vi "Auto Play Path.vi"(7 "PID Constants":T1, 8 "Operation":T2, 9 "Auto Data":T14, 10 "Motors":T3 {"Radii (ft)"."Right Back Position" format="%.2f"; "Radii (ft)"."Right Front Position" format="%.2f"; "Radii (ft)"."Left Back Position" format="%.2f"; "Radii (ft)"."Left Front Position" format="%.2f"; "Pigeon2"."Type" items=["CAN"=352321536, "TalonSRX"=33554432]}) -> (0 "Auto Done?":bool)   [LabVIEW 2023]
uses:
  swerve/Type Definitions/Data/Robot Velocities.ctl
  swerve/Type Definitions/Hardware/Swerve Drives/(NEO-NEO-ThroughBore-Pigeon2) Swerve.ctl
  swerve/Type Definitions/Hardware/4 Motor Sets/(NEO & NEO 550) 4 Motor Set.ctl
  <vilib>/Rock Robotics/WPI/MotorControl/WPI_MotorControlDeviceRef.ctl
  <vilib>/Rock Robotics/WPI/MotorControl/WPI_MotorControlType.ctl
  <vilib>/Rock Robotics/SystemInterfaces/DIO/FPGA_DIOPWMChannel.ctl
  <vilib>/Rock Robotics/WPI/PWM/WPI_PWMDeadband.ctl
  <vilib>/Rock Robotics/SystemInterfaces/DIO/FPGA_DIOChannel.ctl
  <vilib>/Rock Robotics/WPI/ThirdParty/Phoenix-LabVIEW/Pigeon IMU/CTRE_PigeonIMU_DeviceRef.ctl
  <vilib>/Rock Robotics/WPI/ThirdParty/Phoenix-LabVIEW/Pigeon IMU/CTRE_PigeonIMU_ConnectionType.ctl
  swerve/Type Definitions/Data/Pod Positions.ctl
  Implementation/Drive Operations.ctl
  <vilib>/Platform/TimedLoop/XDataNode/timing_clust.ctl
  <vilib>/Platform/TimedLoop/XDataNode/nitl_modes.ctl
  <vilib>/Platform/TimedLoop/XDataNode/wakeup.ctl
  <vilib>/Rock Robotics/WPI/ThirdParty/REV Robotics/REVLib/Typedef/Spark MAX Control Type.ctl
  <vilib>/Rock Robotics/WPI/DriverStation/WPI_DriverStationRobotMode2.ctl
  c1434f1d-cc94-402a-bfa5-996335562ac8.vi
  Framework/Robot Global Data.vi
  <vilib>/Platform/TimedLoop/XDataNode/XDataNode.xnode
  <vilib>/Platform/TimedLoop/XDataNode/XDNodeRunTimeDep.lvlib
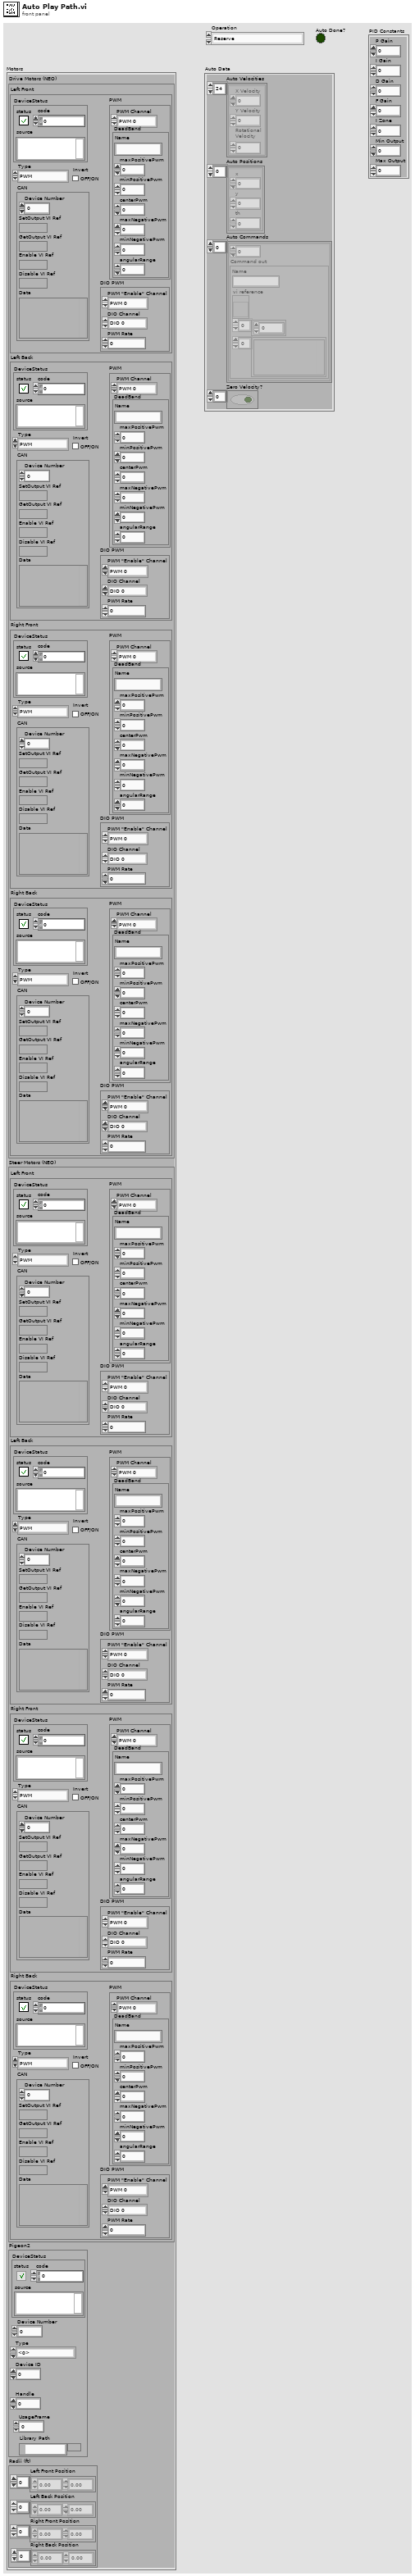
[diagram p1: front panel]
types:
  T1 = cluster{"P Gain":dbl, "I Gain":dbl, "D Gain":dbl, "F Gain":dbl, "I Zone":dbl, "Min Output":dbl, "Max Output":dbl}
  T2 = typedef "Drive Operations.ctl" = enum16{"Reserve", "Read Current", "Immediate", "Calibrate", "Reef Align", "Auto", "Old Reef Align"}
  T3 = typedef "(NEO-NEO-ThroughBore-Pigeon2) Swerve.ctl" = cluster{"Drive Motors (NEO)":T4, "Steer Motors (NEO)":T4, "Pigeon2":T10, "Radii (ft)":T12}
  T4 = typedef "(NEO & NEO 550) 4 Motor Set.ctl" = cluster{"Left Front":T5, "Left Back":T5, "Right Front":T5, "Right Back":T5}
  T5 = typedef "WPI_MotorControlDeviceRef.ctl" = cluster{"DeviceStatus":errorcluster, "Type":T6, "PWM":cluster{"PWM Channel":T7, "DeadBand":T8}, "CAN":cluster{"Device Number":u8, "SetOutput VI Ref":variant, "GetOutput VI Ref":variant, "Enable VI Ref":variant, "Disable VI Ref":variant, "Data":variant}, "Invert":bool, "DIO PWM":cluster{"PWM \"Enable\" Channel":T7, "DIOChannel":T9, "PWM Rate":dbl}}
  T6 = typedef "WPI_MotorControlType.ctl" = enum16{"PWM", "CAN", "DIO PWM"}
  T7 = typedef "FPGA_DIOPWMChannel.ctl" = enum8{"PWM 0", "PWM 1", "PWM 2", "PWM 3", "PWM 4", "PWM 5", "PWM 6", "PWM 7", "PWM 8", "PWM 9", "PWM MXP 0", "PWM MXP 1", "PWM MXP 2", "PWM MXP 3", "PWM MXP 4", "PWM MXP 5", "PWM MXP 6", "PWM MXP 7", "PWM MXP 8", "PWM MXP 9", "Invalid"}
  T8 = typedef "WPI_PWMDeadband.ctl" = cluster{"Name":string, "maxPositivePwm":i32, "minPositivePwm":i32, "centerPwm":i32, "maxNegativePwm":i32, "minNegativePwm":i32, "angularRange":u16}
  T9 = typedef "FPGA_DIOChannel.ctl" = enum8{"DIO 0", "DIO 1", "DIO 2", "DIO 3", "DIO 4", "DIO 5", "DIO 6", "DIO 7", "DIO 8", "DIO 9", "DIO MXP 0", "DIO MXP 1", "DIO MXP 2", "DIO MXP 3", "DIO MXP 4", "DIO MXP 5", "DIO MXP 6", "DIO MXP 7", "DIO MXP 8", "DIO MXP 9", "DIO MXP 10", "DIO MXP 11", "DIO MXP 12", "DIO MXP 13", "DIO MXP 14", "DIO MXP 15", "SPI Port CS1", "SPI Port CS2", "SPI Port CS3", "SPI Port MISO", "SPI Port MOSI", "Invalid"}
  T10 = typedef "CTRE_PigeonIMU_DeviceRef.ctl" = cluster{"DeviceStatus":errorcluster, "Device Number":u8, "Type":T11, "Device ID":u32, "Handle":u64, "UsageFrame":u32, "Library Path":path}
  T11 = typedef "CTRE_PigeonIMU_ConnectionType.ctl" = u32
  T12 = typedef "Pod Positions.ctl" = cluster{"Left Front Position":dbl[], "Left Back Position":dbl[], "Right Front Position":dbl[], "Right Back Position":dbl[]}
  T13 = typedef "Robot Velocities.ctl" = cluster{"X Velocity":dbl, "Y Velocity":dbl, "Rotational \nVelocity":dbl}
  T14 = cluster{"Auto Velocities":T13[], "Auto Positions":cluster{"x":dbl, "y":dbl, "th":dbl}[], "Auto Commands":cluster{dbl, "Command out":cluster{"Name":string, "vi reference":refnum<vi>, i32[], variant[]}}[], "Zero Velocity?":bool[]}
  T15 = cluster{"Time (s)":dbl, "Command out":cluster{"Name":string, "vi reference":refnum<vi>, i32[], variant[]}}
  T16 = typedef "Spark MAX Control Type.ctl" = enum16{"Percent VBus", "Voltage", "Velocity", "Position", "Smart Motion", "Current", "Smart Velocity", "MAXMotion Position", "MAXMotion Velocity"}
  T17 = cluster{"Left Front":dbl, "Left Back":dbl, "Right Front":dbl, "Right Back":dbl}
  T18 = typedef "XDNodeRunTimeDep.lvlib/timing_clust.ctl" = cluster{"Expected End [f-1]":u64, "Actual End [f-1]":u64, "Finished Late? [f-1]":bool, "Expected End [i-1]":u64, "Actual End [i-1]":u64, "Finished Late? [i-1]":bool, "Expected Start [i]":u64, "Actual Start [i]":u64, "Expected Start [f]":u64, "Actual Start [f]":u64, "Source Name":string, "Structure Name":string, "Period":i64, "Deadline":i64, "Offset":i64, "Start":i64, "Priority":i32, "Timeout":i32, "Mode":T19, "Wakeup Reason":T20, "Error":errorcluster, "Source Type":string, "Secondary Source Type":string, "Global End Time":u64, "Global Start Time":u64, "Frame Duration":u64, "Iteration Duration":u64, "Assigned CPU":i32, "I/O Scan Engine Mode":u32}
  T19 = typedef "XDNodeRunTimeDep.lvlib/nitl_modes.ctl" = enum32{"No Change", "Process missed periods, maintain original phase", "Discard missed periods, maintain original phase", "Process missed periods, ignore original phase", "Discard missed periods, ignore original phase"}
  T20 = typedef "XDNodeRunTimeDep.lvlib/wakeup.ctl" = enum32{"Normal", "Aborted", "Asynchronous wakeup", "Timing source error", "Timed loop error", "Timeout"}
  T21 = cluster{dbl, "Command out":cluster{"Name":string, "vi reference":refnum<vi>, i32[], variant[]}}[]
  T22 = typedef "WPI_DriverStationRobotMode2.ctl" = enum16{"Autonomous Disabled", "Autonomous Enabled", "Teleop Disabled", "Teleop Enabled", "Disconnected", "Finish", "Test Disabled", "Test Enabled", "Emergency Stopped"}
  T23 = cluster{"Field Centric":bool, "Reef Centric":bool}
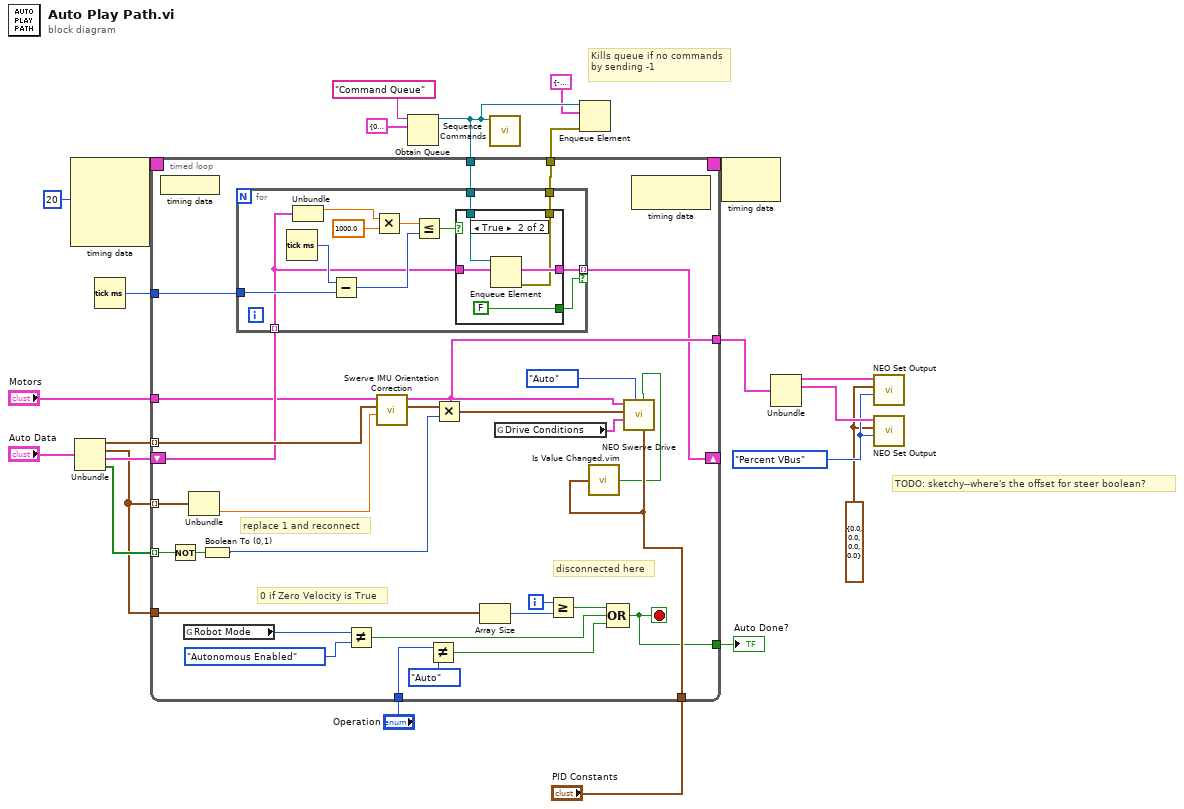
[diagram p0: block diagram]
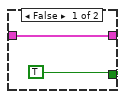
[diagram p2: hidden frame]
diagram:
  w8 = Spark_MAX_Control_Type."Percent VBus" ("Control Mode")
  w7 = T17 {"Left Front"=0.0, "Left Back"=0.0, "Right Front"=0.0, "Right Back"=0.0} ("Setpoints")
  # "TODO: sketchy--where's the offset for steer boolean?"
  # "Kills queue if no commands by sending -1"
  n1 = node-c288(i64 20 ("Period")) -> (w23:T18)  [unwired: 3 in]
  n2 = Unbundle("Auto Data") -> ("Auto Velocities"=w16:T13[], "Auto Positions"=w17:cluster{"x":dbl, "y":dbl, "th":dbl}[], "Auto Commands"=w19:T21, "Zero Velocity?"=w20:bool[])
  n3 = Tick Count (ms)() -> (millisecond timer value=w18:u32)
  n4 = Obtain Queue(name (unnamed)="Command Queue", element data type=T15 {"Time (s)"=0.0, "Command out"={"Name"="", "vi reference"=refnum, [], []}} ("element")) -> (queue out=w4:refnum<queue>)  [unwired: 3 in, 2 out]
  n5 = timed-loop {
    timing: w23 -> [_]
    timing-out: [_] -> w22
    tunnel: "Motors" -> [w39]
    tunnel: [w51] -> w6
    tunnel: w16 -> [w50] mode=indexing
    tunnel: w17 -> [w49] mode=indexing
    tunnel: w17 -> [w48]
    tunnel: w18 -> [w47]
    tunnel: w4 -> [w46]
    shift-right: [w45] -> _
    shift-left: w19 -> [w44]
    tunnel: w20 -> [w40] mode=indexing
    tunnel: [w29] -> w21
    tunnel: "Operation" -> [w38]
    tunnel: [w37] -> w3
    tunnel: "PID Constants" -> [w34]
    i -> [w52]
    stop <- w29 stop-if-true
    # "replace 1 and reconnect"
    # "disconnected here"
    # "0 if Zero Velocity is True"
    n6 = node-c288() -> ()  [unwired: 1 in]
    n7 = Not(x=w40) -> (.not. x?=w28:bool)
    n8 = global read "Robot Global Data.vi" "Robot Mode"() -> (w33:T22)
    n9 = Unbundle(w49) -> ("th"=w35:dbl)  [unwired: 2 out]
    n10 = Boolean To (0,1)(Boolean=w28) -> (0, 1=w27:i16)
    n11 = for {
      tunnel: w47 -> [w64]
      tunnel: w46 -> [w58]
      tunnel: w44 -> [w55] mode=indexing
      tunnel: [w57] -> w45 mode=indexing if=w56
      tunnel: [w54] -> w37
      n12 = Tick Count (ms)() -> (millisecond timer value=w65:u32)
      n13 = Unbundle(w55) -> (w63:dbl)  [unwired: 1 out]
      n14 = Subtract(x=w65, y=w64) -> (x-y=w60:u32)
      n15 = Multiply(x=w63, y=1000.0) -> (x*y=w61:dbl)
      n16 = Less Or Equal?(x=w61, y=w60) -> (x <= y?=w59:bool)
      n17 = case shown="True" w59 {
        tunnel: w58 -> [_ w71]
        tunnel: w55 -> [w66 w70]
        tunnel: [w66 w70] -> w57
        tunnel: [TRUE FALSE] -> w56
        tunnel: [_ w68] -> w54
        frame False {
        }
        frame True {
          n18 = Enqueue Element(queue=w71, element=w70) -> (error out=w68:errorcluster)  [unwired: 2 in, 2 out]
        }
      }
    }
    n19 = Not Equal?(x=w33, y=WPI_DriverStationRobotMode2."Autonomous Enabled") -> (x != y?=w42:bool)
    n20 = call "Swerve IMU Orientation Correction.vi"("Setpoint"=w35, "Robot Velocities In"=w50, "Motors In"=w39) -> ("Robot Velocities Out"=w36:T13, "Motors Out"=w51:T3)  [unwired: 7 in]
    n21 = Not Equal?(x=w38, y=Drive_Operations."Auto") -> (x != y?=w41:bool)
    n22 = Multiply(x=w36, y=w27) -> (x*y=w43:T13)
    n23 = Array Size(array=w48) -> (size(s)=w53:i32)
    n24 = global read "Robot Global Data.vi" "Drive Conditions"() -> (w25:T23)
    n25 = Greater Or Equal?(x=w52, y=w53) -> (x >= y?=w30:bool)
    n26 = call "Is Value Changed.vim"("value"=w34) -> ("changed or first call?"=w24:bool)
    n27 = Compound Arithmetic op=OR(w30, w42, w41) -> (w29:bool)
    n28 = call "NEO Swerve Drive.vi"("PID Constants"=w34, "Configure?"=w24, "Operation"=Drive_Operations."Auto", "Drive Conditions"=w25, "Robot Velocities"=w43, "Swerve Drive"=w51) -> ()  [unwired: 5 in, 1 out]
    n29 = node-c288() -> ()  [unwired: 1 in, 1 out]
  }
  "Auto Done?" <- w21
  n30 = call "Sequence Commands.vi"("queue in"=w4) -> ()  [unwired: 11 in]
  n31 = Enqueue Element(queue=w4, element=T15 {"Time (s)"=-1.0, "Command out"={"Name"="", "vi reference"=refnum, [], []}}, error in (no error)=w3) -> ()  [unwired: 1 in, 3 out]
  n32 = node-c288(w22) -> ()  [unwired: 1 out]
  n33 = Unbundle(w6) -> ("Drive Motors (NEO)"=w10:T4, "Steer Motors (NEO)"=w9:T4)  [unwired: 2 out]
  n34 = call "NEO Set Output.vi"("Control Mode"=w8, "Setpoints"=w7, "Motors"=w10) -> ()  [unwired: 9 in]
  n35 = call "NEO Set Output.vi"("Control Mode"=w8, "Setpoints"=w7, "Motors"=w9) -> ()  [unwired: 9 in]
